vi "ParseMermaidString.vi"(8 "error in (no error)":errorcluster, 11 "ParseMermaid in":refnum<class "ParseMermaid.lvclass">) -> (0 "error out":errorcluster, 3 "ParseMermaid out":refnum<class "ParseMermaid.lvclass">)   [LabVIEW 2020, in "Mermaid.lvlib" / "ParseMermaid.lvclass"]
uses:
  ParseMermaid.lvclass
  ParseMermaid.lvclass/ParseMermaid.ctl
  <vilib>/regexp/Match Regular Expression.xnode
panel:
  out "Title":string
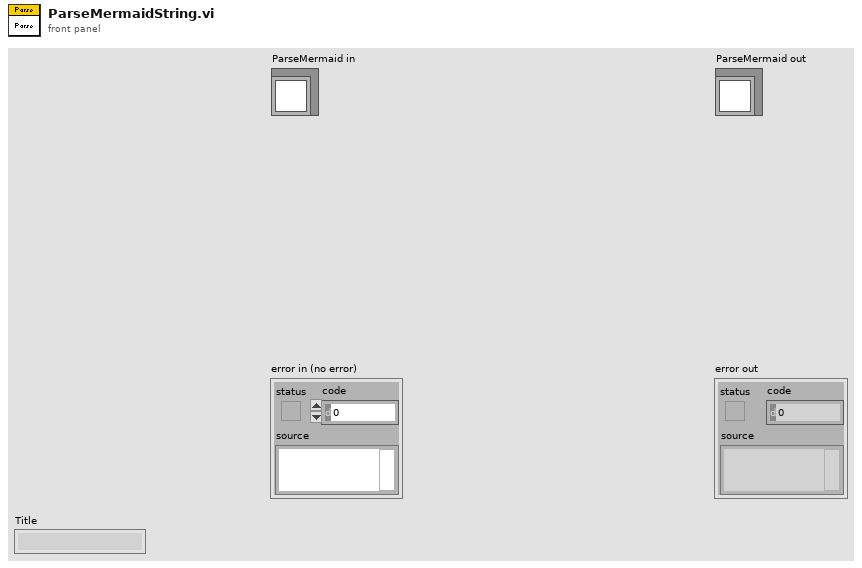
[diagram p1: front panel]
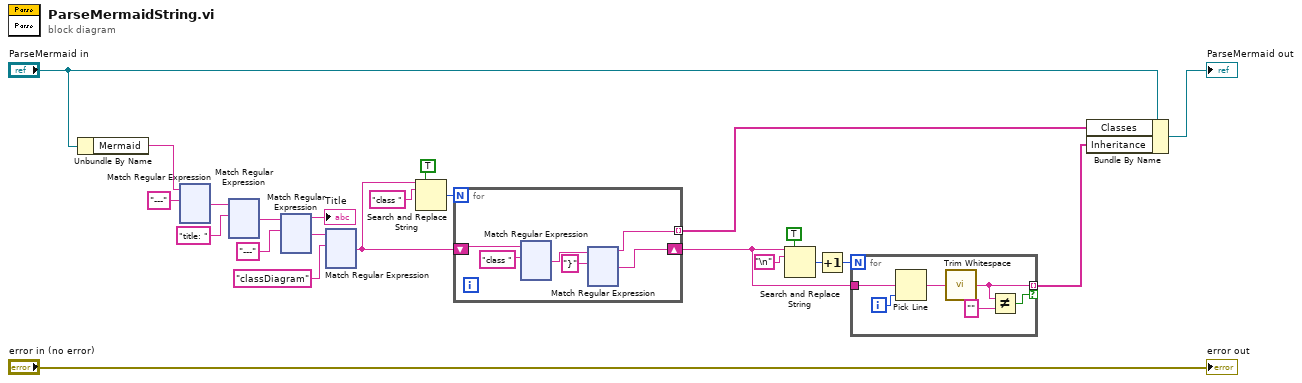
[diagram p0: block diagram]
diagram:
  n1 = Unbundle By Name("ParseMermaid in") -> ("Mermaid"=w5:string)
  n2 = xnode "Match Regular Expression"("input string"=w5, "regular expression"="---") -> ("after match"=w21:string)  [unwired: 4 in, 4 out]
  n3 = xnode "Match Regular Expression"("input string"=w21, "regular expression"="title: ") -> ("after match"=w18:string)  [unwired: 4 in, 4 out]
  n4 = xnode "Match Regular Expression"("input string"=w18, "regular expression"="---") -> ("before match"=→"Title":string, "after match"=w16:string)  [unwired: 4 in, 3 out]
  n5 = xnode "Match Regular Expression"("input string"=w16, "regular expression"="classDiagram") -> ("after match"=w14:string)  [unwired: 4 in, 4 out]
  n6 = Search and Replace String(replace all?=TRUE ("replace all? (F)"), input string=w14, search string="class " ("regular expression")) -> (number of replacements=w12:i32)  [unwired: 5 in, 3 out]
  n7 = for {
    N: w12 -> [_]
    shift-right: [w24] -> w7
    shift-left: w14 -> [w26]
    tunnel: [w25] -> w2 mode=indexing
    n8 = xnode "Match Regular Expression"("input string"=w26, "regular expression"="class ") -> ("after match"=w28:string)  [unwired: 4 in, 4 out]
    n9 = xnode "Match Regular Expression"("input string"=w28, "regular expression"="}") -> ("before match"=w25:string, "after match"=w24:string)  [unwired: 4 in, 3 out]
  }
  n10 = Search and Replace String(replace all?=TRUE ("replace all? (F)"), input string=w7, search string="\n") -> (number of replacements=w8:i32)  [unwired: 5 in, 3 out]
  n11 = Increment(x=w8) -> (x+1=w6:i32)
  n12 = for {
    N: w6 -> [_]
    tunnel: w7 -> [w263]
    tunnel: [w258] -> w1 mode=indexing if=w260
    i -> [w262]
    n13 = Pick Line(multi-line string=w263, line index=w262) -> (output string=w259:string)  [unwired: 1 in]
    n14 = call <vilib>:"Trim Whitespace.vi"("string"=w259) -> ("trimmed string"=w258:string)  [unwired: 1 in]
    n15 = Not Equal?(x=w258, y="") -> (x != y?=w260:bool)
  }
  n16 = Bundle By Name(cluster="ParseMermaid in", "Classes"=w2, "Inheritance"=w1) -> (→"ParseMermaid out":refnum<class "ParseMermaid.lvclass">)
  "error out" <- "error in (no error)"
